vi "ADIS16448 Scale Data.vi"(8 "error in (no error)":errorcluster, 10 "New Data In":u8[](array[numeric])) -> (0 "error out":errorcluster, 1 "Data Good?":bool, 2 "Data Out":dbl[](array[numeric]), 3 "output cluster":T1)   [LabVIEW 2025]
uses:
  <vilib>/Rock Robotics/WPI/ThirdParty/ADI/ADIS16448/Typedef/ADIS16448 Data.ctl
panel:
  in  "element":T1
  out "Calculated CRC-16":u16
  out "Received CRC-16":u16
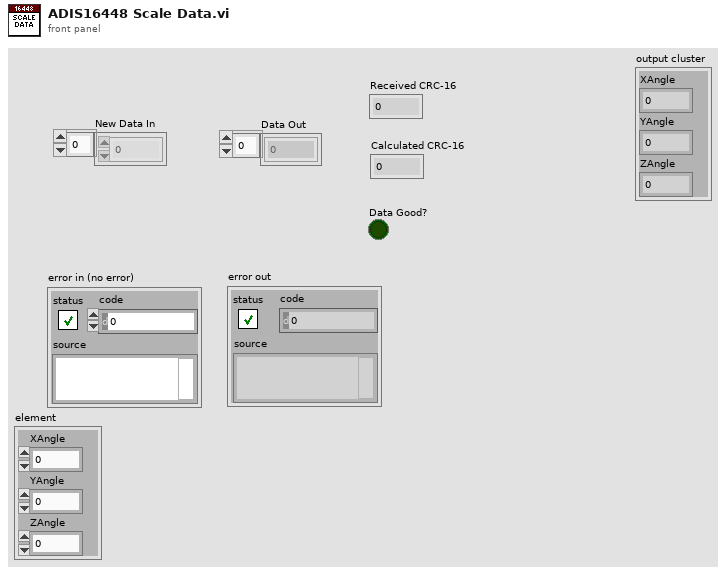
[diagram p1: front panel]
types:
  T1 = typedef "ADIS16448 Data.ctl" = cluster{"XAngle":dbl, "YAngle":dbl, "ZAngle":dbl}
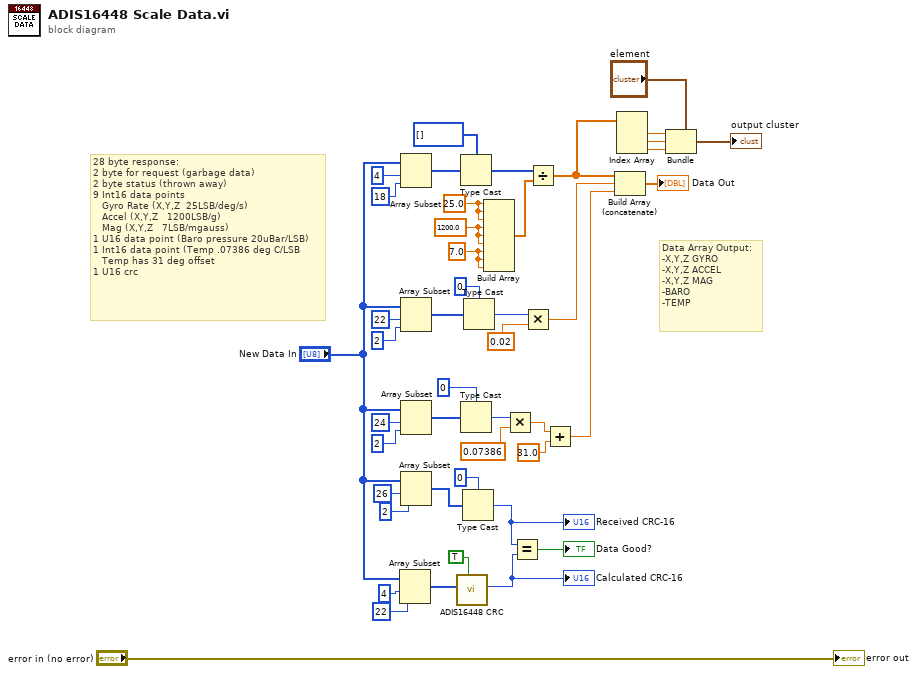
[diagram p0: block diagram]
diagram:
  w43 = 7.0
  w44 = 1200.0
  w45 = 25.0 ("element")
  # "Data Array Output:\n-X,Y,Z GYRO\n-X,Y,Z ACCEL\n-X,Y,Z MAG\n-BARO\n-TEMP"
  # "28 byte response:\n2 byte for request (garbage data)\n2 byte status (thrown away)\n9 Int16 data points\n   Gyro Rate (X,Y,Z  25LSB/deg/s)\n   Accel (X,Y,Z   1200LSB/g)\n   Mag (X,Y,Z   7LSB/mgauss)\n1 U16 data point (Baro pressure 20uBar/LSB)\n1 Int16 data point (Temp .07386 deg C/LSB\n   Temp has 31 deg offset\n1 U16 crc"
  n1 = Array Subset(array="New Data In", index=4, length=22) -> (w11:u8[])
  n2 = Array Subset(array="New Data In", index=4, length=18) -> (w23:u8[])
  n3 = Array Subset(array="New Data In", index=22, length=2) -> (w29:u8[])
  n4 = Array Subset(array="New Data In", index=24, length=2) -> (w27:u8[])
  n5 = Array Subset(array="New Data In", index=26, length=2) -> (w17:u8[])
  n6 = call <vilib>:"ADIS16448 CRC.vi"("Look-Up Table Method?"=TRUE, "Byte Array (MSB-First)"=w11) -> ("CRC16-ADIS"=w10:u16)  [unwired: 9 in]
  "Calculated CRC-16" <- w10
  n7 = Type Cast(type=i16[] [], x=w23) -> (*(type *) &x=w22:i16[])
  n8 = Type Cast(type=i16 0, x=w27) -> (*(type *) &x=w24:i16)
  n9 = Type Cast(type=u16 0, x=w17) -> (*(type *) &x=w14:u16)
  "Received CRC-16" <- w14
  n10 = Type Cast(type=u16 0, x=w29) -> (*(type *) &x=w25:u16)
  n11 = Build Array(w45, w45, w45, w44, w44, w44, w43, w43, w43) -> (w42:dbl[])
  n12 = Multiply(x=w24, y=0.07386 ("element")) -> (x*y=w39:dbl)
  n13 = Equal?(x=w14, y=w10) -> (x = y?=→"Data Good?":bool)
  n14 = Multiply(x=w25, y=0.02) -> (x*y=w36:dbl)
  n15 = Divide(x=w22, y=w42) -> (x/y=w6:dbl[])
  n16 = Add(x=w39, y=31.0) -> (x+y=w37:dbl)
  n17 = Build Array (concatenate)(w6, w36, w37) -> (→"Data Out":dbl[])
  n18 = Index Array(array=w6) -> (element #1=w5:dbl, element #2=w4:dbl, element #3=w3:dbl)  [unwired: 3 in]
  n19 = Bundle(cluster="element", "XAngle"=w5, "YAngle"=w4, "ZAngle"=w3) -> (→"output cluster":T1)
  "error out" <- "error in (no error)"
